vi "Read Remote Terminals.vi"(8 "error in":errorcluster, 11 "port in":T1 format="%.0x") -> (0 "error out":errorcluster, 1 "terminal names":string[](array[string]), 2 "terminals":T2[](array[typedef]), 3 "port out":T1 format="%.0x")   [LabVIEW 2020, in "Ballard MIL-STD-1553 Scripting.lvlib"]
uses:
  Ballard MIL-STD-1553 Scripting.lvlib
  Shared/Address.ctl
  <vilib>/NI VeriStand/Custom Device API/Custom Device Item Ref.ctl
  <vilib>/NI VeriStand/Custom Device API/Custom Device API.lvlib
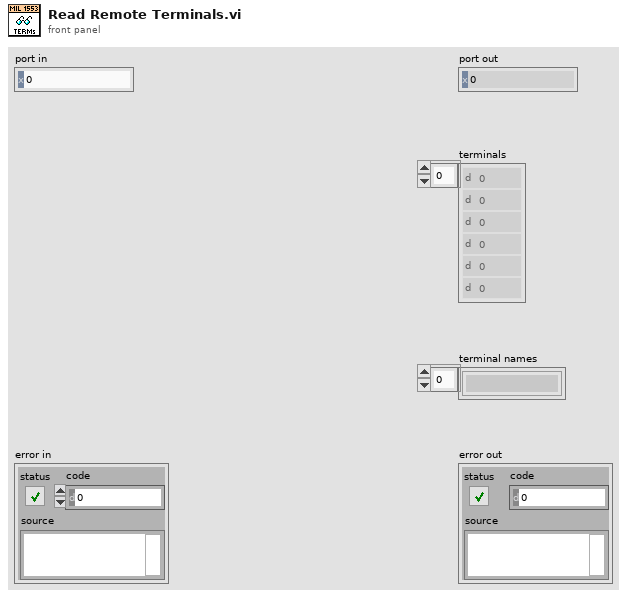
[diagram p1: front panel]
types:
  T1 = typedef "Custom Device API.lvlib/Custom Device Item Ref.ctl" = u64
  T2 = typedef "Address.ctl" = u16
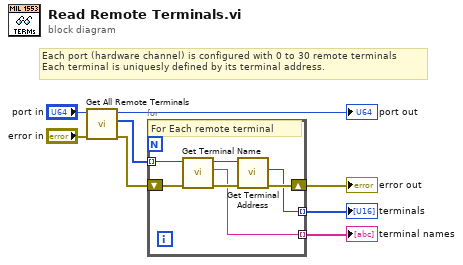
[diagram p0: block diagram]
diagram:
  # "Each port (hardware channel) is configured with 0 to 30 remote terminals\nEach terminal is uniquesly defined by its terminal address."
  n1 = call "Get All Remote Terminals.vi"("error in"="error in", "port in"="port in") -> ("error out"=w3:errorcluster, "remote terminals"=w4:T1[], "port out"=→"port out":T1)  [unwired: 7 in]
  n2 = for {
    shift-right: [w15] -> w8
    shift-left: w3 -> [w11]
    tunnel: w4 -> [w12] mode=indexing
    tunnel: [w14] -> w2 mode=indexing
    tunnel: [w9] -> w1 mode=indexing
    # "For Each remote terminal"
    n3 = call "Get Terminal Name.vi"("error in"=w11, "remote terminal in"=w12) -> ("error out"=w10:errorcluster, "terminal name"=w9:string, "remote terminal out"=w13:T1)  [unwired: 7 in]
    n4 = call "Get Terminal Address.vi"("error in"=w10, "remote terminal in"=w13) -> ("error out"=w15:errorcluster, "terminal address"=w14:T2)  [unwired: 6 in, 2 out]
  }
  "error out" <- w8
  "terminals" <- w2
  "terminal names" <- w1
